vi "Global_Init.vi"(11 "Object":T1) -> ()   [LabVIEW 2020]
uses:
  <resource>/Framework/Providers/API/ItemRef.ctl
  <resource>/Framework/Providers/API/mxLvMenuItem.ctl
panel:
  out "error out":errorcluster
  in  "error in":errorcluster
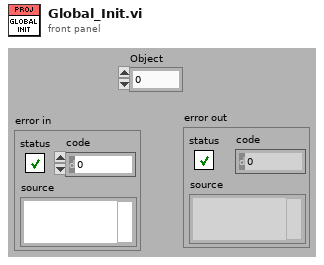
[diagram p1: front panel]
types:
  T1 = typedef "ItemRef.ctl" = u64
  T2 = typedef "mxLvMenuItem.ctl" = cluster{"Menu Name":string, "Description":string, "Icon File Name":path, "Menu Tag":string, "Enabled":bool, "Checked":bool, "Separator":bool, "Batchable":bool, "Weight":i32, "Batch Mode (Ignored if Not Batchable)":enum32{"Show If All Items Support Command", "Show If Any Items Support Command"}, "Menu Location":enum32{"<None>", "Project", "Project / Build Specifications", "Tools", "Tools / Source Control", "Tools / Real-Time Module", "Help"}, "Exclude From Getting Started Window Menu":bool}
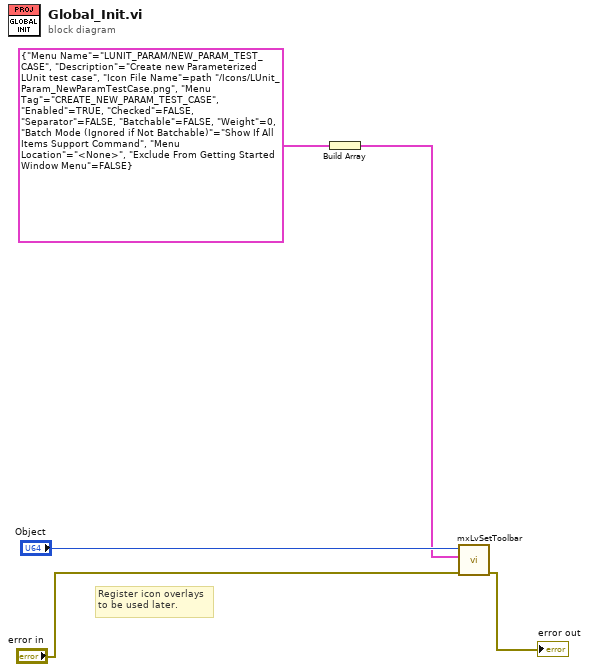
[diagram p0: block diagram]
diagram:
  # "Register icon overlays\nto be used later."
  n1 = Build Array(T2 {"Menu Name"="LUNIT_PARAM/NEW_PARAM_TEST_CASE", "Description"="Create new Parameterized LUnit test case", "Icon File Name"=path "../Icons/LUnit_Param_NewParamTestCase.png", "Menu Tag"="CREATE_NEW_PARAM_TEST_CASE", "Enabled"=TRUE, "Checked"=FALSE, "Separator"=FALSE, "Batchable"=FALSE, "Weight"=0, "Batch Mode (Ignored if Not Batchable)"=enum."Show If All Items Support Command", "Menu Location"=enum."<None>", "Exclude From Getting Started Window Menu"=FALSE} ("Menu Item")) -> (w2:T2[])
  n2 = call <resource>:"mxLvSetToolbar.vi"("error in"="error in", "Toolbar Items"=w2, "Item"="Object") -> ("error out"=→"error out":errorcluster)  [unwired: 7 in, 1 out]
